vi "ASM.Event.Error.vi"(8 "error in (no error)":errorcluster, 10 "StateError":errorcluster, 11 "ActorStateMachine in":refnum<class "ActorStateMachine.lvclass">) -> (0 "error out":errorcluster, 3 "ActorStateMachine out":refnum<class "ActorStateMachine.lvclass">)   [LabVIEW 2021, in "ActorStateMachine.lvlib" / "ActorStateMachine.lvclass"]
uses:
  ActorStateMachine.lvclass
  ActorStateMachine.lvclass/ActorStateMachine.ctl
  _ASM.State.ctl
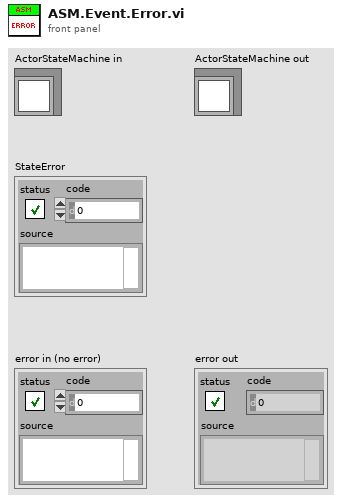
[diagram p1: front panel]
types:
  T1 = typedef "ActorStateMachine.lvlib/ActorStateMachine.lvclass/_ASM.State.ctl" = enum16{"Boom", "Pre-Init", "Init", "Post-Init", "Pre-Reset", "Reset", "Post-Reset", "Pre-Config", "Config", "Post-Config", "Pre-Ready", "Ready", "Post-Ready", "Pre-Running", "Running", "Next", "Post-Running", "Break", "Fail", "Crash", "Shutdown", "Doom"}
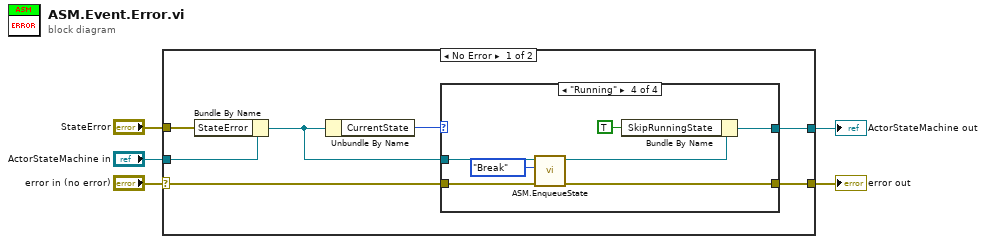
[diagram p0: block diagram]
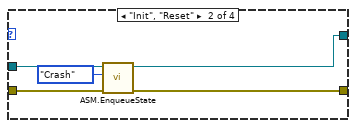
[diagram p3: hidden frame]
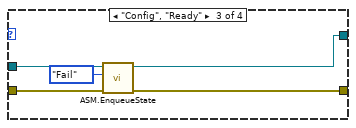
[diagram p4: hidden frame]
diagram:
  n1 = case shown="No Error" "error in (no error)" {
    selector: "error in (no error)" -> [w11 w33]
    tunnel: [w10 w33] -> w4
    tunnel: [w9 w32] -> w2
    tunnel: "ActorStateMachine in" -> [w6 w32]
    tunnel: "StateError" -> [w8 _]
    frame No Error {
      n2 = Bundle By Name(cluster=w6, "StateError"=w8) -> (w7:refnum<class "ActorStateMachine.lvclass">)
      n3 = Unbundle By Name(w7) -> ("CurrentState"=w12:T1)
      n4 = case shown="\"Running\"" w12 {
        tunnel: w11 -> [w13 w19 w24 w31]
        tunnel: [w13 w18 w23 w30] -> w10
        tunnel: w7 -> [w14 w17 w22 w29]
        tunnel: [w14 w15 w20 w26] -> w9
        frame Default {
        }
        frame "Init", "Reset" {
          n5 = call "ASM.EnqueueState.vi"("error in (no error)"=w19, "NextState"=_ASM.State."Crash", "ActorStateMachine in"=w17) -> ("error out"=w18:errorcluster, "ActorStateMachine out"=w15:refnum<class "ActorStateMachine.lvclass">)  [unwired: 7 in]
        }
        frame "Config", "Ready" {
          n6 = call "ASM.EnqueueState.vi"("error in (no error)"=w24, "NextState"=_ASM.State."Fail", "ActorStateMachine in"=w22) -> ("error out"=w23:errorcluster, "ActorStateMachine out"=w20:refnum<class "ActorStateMachine.lvclass">)  [unwired: 7 in]
        }
        frame "Running" {
          n7 = call "ASM.EnqueueState.vi"("error in (no error)"=w31, "NextState"=_ASM.State."Break", "ActorStateMachine in"=w29) -> ("error out"=w30:errorcluster, "ActorStateMachine out"=w27:refnum<class "ActorStateMachine.lvclass">)  [unwired: 7 in]
          n8 = Bundle By Name(cluster=w27, "SkipRunningState"=TRUE) -> (w26:refnum<class "ActorStateMachine.lvclass">)
        }
      }
    }
    frame Error {
    }
  }
  "error out" <- w4
  "ActorStateMachine out" <- w2
